vi "Kalman F.vi"(10 "Ball?":bool, 11 "intervalo":dbl) -> (1 "Q":T1, 2 "F'":T1, 3 "F":T1)   [LabVIEW 2017]
uses:
  <vilib>/Analysis/Matrix/Datatypes/RealMatrix.ctl
  <vilib>/Analysis/Matrix/Numeric/Multiply/Multiply - R,RM.vi
  <vilib>/Analysis/Matrix/Numeric/Add/Add - RM,RM.vi
  <vilib>/Analysis/Matrix/NI_Matrix.lvlib
  <vilib>/Analysis/Matrix/Numeric/Multiply/Multiply - RM,RM.vi
  <vilib>/Analysis/Matrix/Numeric/Conversions/Array To Matrix - RA2.vi
  <vilib>/Analysis/Matrix/Numeric/Conversions/Array To Matrix - RA.vi
  <vilib>/Analysis/Matrix/Numeric/Multiply/Multiply - RM,R.vi
panel:
  out "Real Matrix (Column Vector)":T1
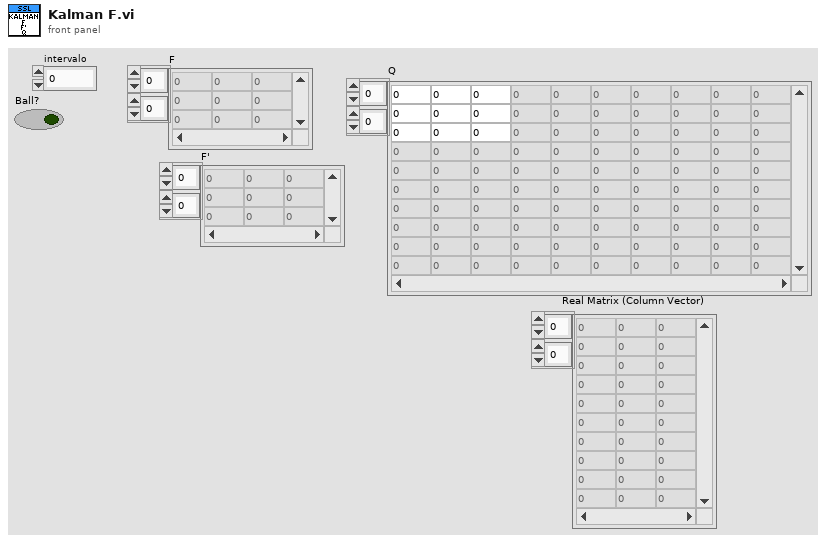
[diagram p1: front panel]
types:
  T1 = typedef "NI_Matrix.lvlib/RealMatrix.ctl" = dbl[][]
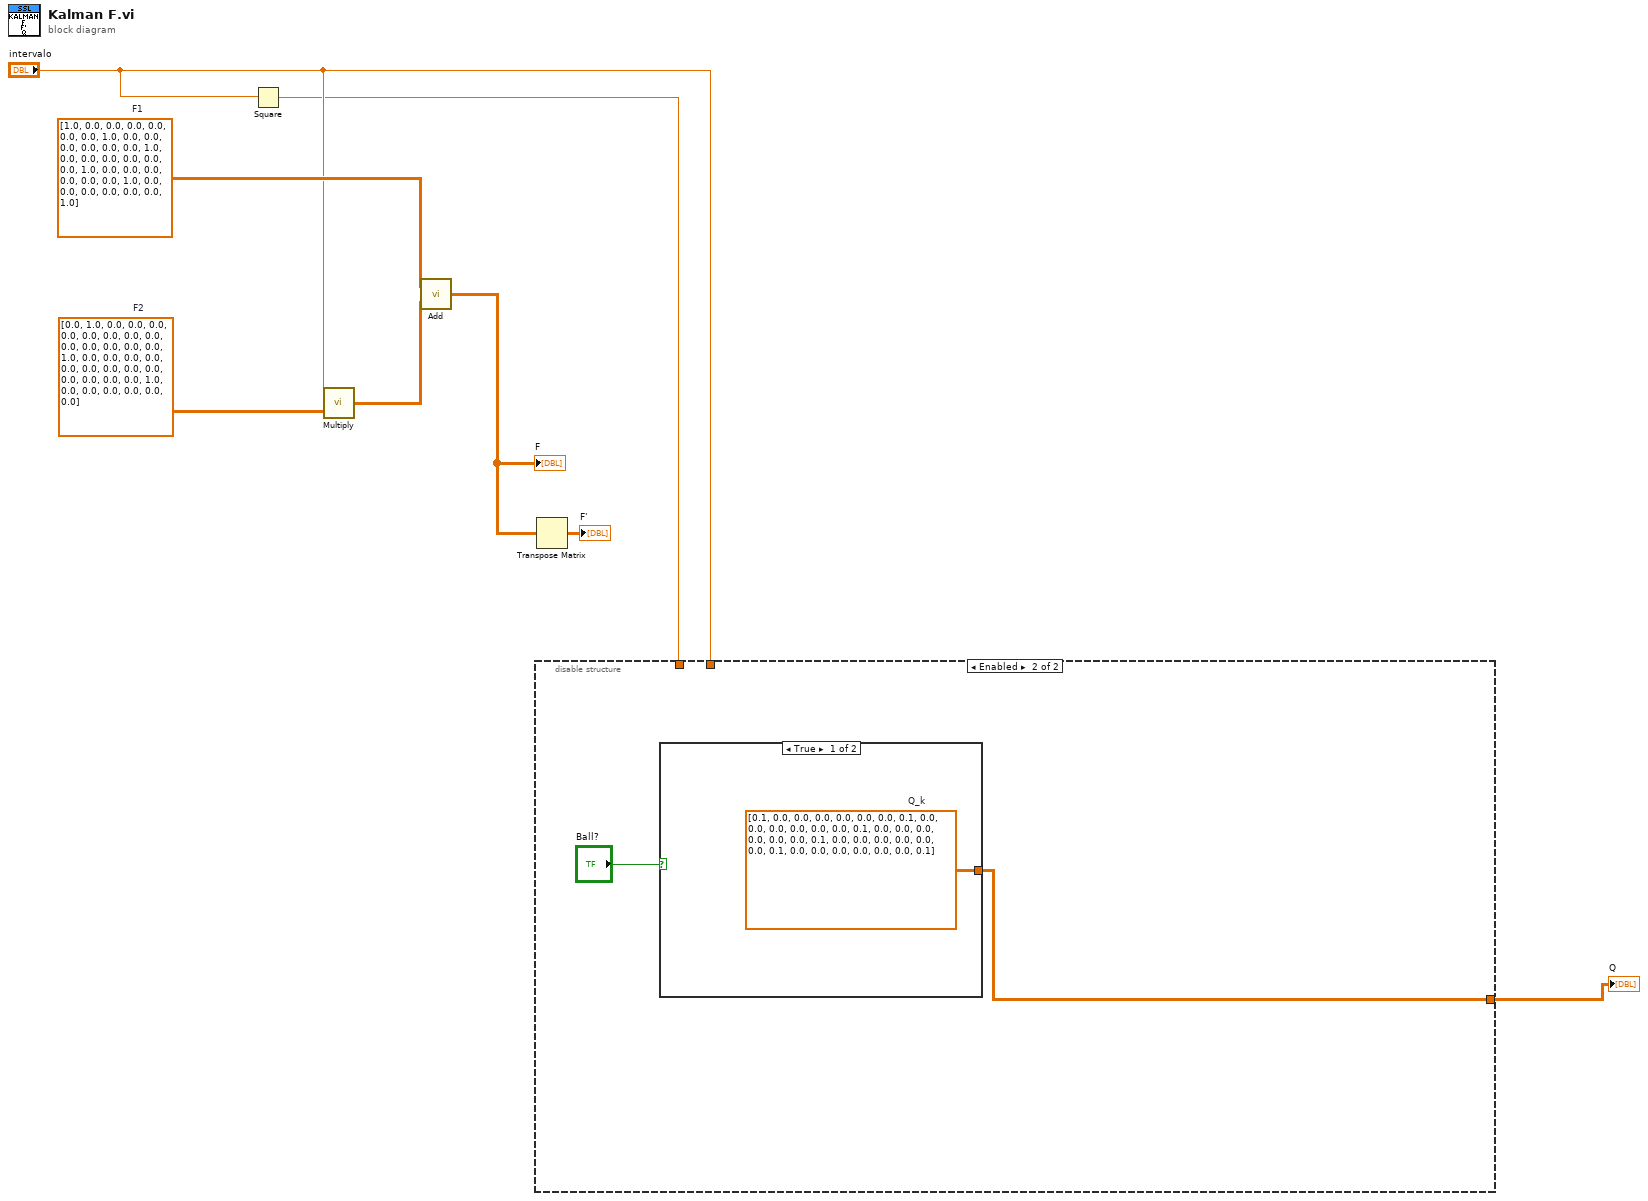
[diagram p0: block diagram]
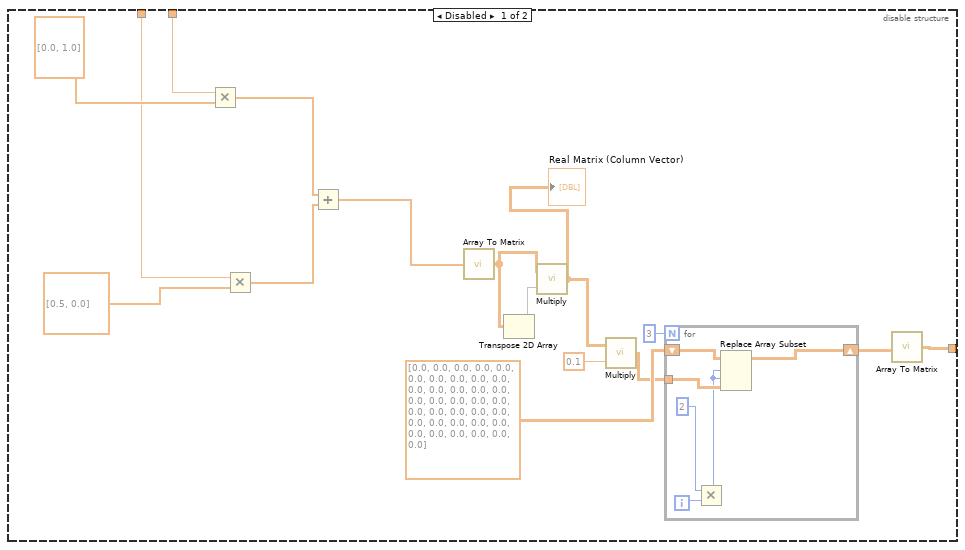
[diagram p2: hidden frame]
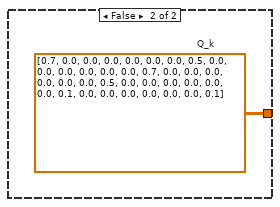
[diagram p3: hidden frame]
diagram:
  w6 = T1 [[0.0, 1.0, 0.0, 0.0, 0.0, 0.0], [0.0, 0.0, 0.0, 0.0, 0.0, 0.0], [0.0, 0.0, 0.0, 1.0, 0.0, 0.0], [0.0, 0.0, 0.0, 0.0, 0.0, 0.0], [0.0, 0.0, 0.0, 0.0, 0.0, 1.0], [0.0, 0.0, 0.0, 0.0, 0.0, 0.0]]  # F2
  w7 = T1 [[1.0, 0.0, 0.0, 0.0, 0.0, 0.0], [0.0, 1.0, 0.0, 0.0, 0.0, 0.0], [0.0, 0.0, 1.0, 0.0, 0.0, 0.0], [0.0, 0.0, 0.0, 1.0, 0.0, 0.0], [0.0, 0.0, 0.0, 0.0, 1.0, 0.0], [0.0, 0.0, 0.0, 0.0, 0.0, 1.0]]  # F1
  n1 = Square(x="intervalo") -> (x^2=w3:dbl)
  n2 = call-poly <vilib>:"Multiply.vi"("Real Matrix A"=w6, "Real Scalar c"="intervalo") -> ("c * A"=w8:T1)
  n3 = call-poly <vilib>:"Add.vi"("Real Matrix B"=w8, "Real Matrix A"=w7) -> ("A + B"=w2:T1)
  "F" <- w2
  n4 = disable-structure shown="Enabled" {
    disable-tunnel: "intervalo" -> [w24 _]
    disable-tunnel: w3 -> [w22 _]
    disable-tunnel: [w12 w32] -> w1
    frame Disabled {
      n5 = Multiply ("Multiply.vi")(x=w24, y=dbl[] [0.0, 1.0]) -> (x*y=w20:dbl[])
      n6 = Multiply ("Multiply.vi")(x=w22, y=dbl[] [0.5, 0.0]) -> (x*y=w19:dbl[])
      n7 = Add(x=w20, y=w19) -> (x+y=w18:dbl[])
      n8 = call-poly <vilib>:"Array To Matrix.vi"("Real 1D Array"=w18) -> ("Real Matrix (Column Vector)"=w16:T1)
      n9 = Transpose 2D Array(2D array=w16) -> (transposed array=w17:T1)
      n10 = call-poly <vilib>:"Multiply.vi"("Real Matrix B"=w17, "Real Matrix A"=w16) -> ("A * B"=w11:T1)
      "Real Matrix (Column Vector)" <- w11
      n11 = call-poly <vilib>:"Multiply.vi"("Real Scalar c"=0.1 ("y"), "Real Matrix A"=w11) -> ("A * c"=w10:T1)
      n12 = for {
        N: 3 -> [_]
        tunnel: w10 -> [w28]
        shift-right: [w27] -> w13
        shift-left: dbl[][] [[0.0, 0.0, 0.0, 0.0, 0.0, 0.0], [0.0, 0.0, 0.0, 0.0, 0.0, 0.0], [0.0, 0.0, 0.0, 0.0, 0.0, 0.0], [0.0, 0.0, 0.0, 0.0, 0.0, 0.0], [0.0, 0.0, 0.0, 0.0, 0.0, 0.0], [0.0, 0.0, 0.0, 0.0, 0.0, 0.0]] -> [w26]
        i -> [w30]
        n13 = Multiply(x=2, y=w30) -> (x*y=w25:i32)
        n14 = Replace Array Subset(array=w26, new element=w28, index (row)=w25, index (col)=w25) -> (w27:dbl[][])
      }
      n15 = call-poly <vilib>:"Array To Matrix.vi"("Real 2D Array"=w13) -> ("Real Matrix"=w12:T1)
    }
    frame Enabled {
      n16 = case shown="True" "Ball?" {
        tunnel: [w33 w34] -> w32
        frame True {
          w33 = T1 [[0.1, 0.0, 0.0, 0.0, 0.0, 0.0], [0.0, 0.1, 0.0, 0.0, 0.0, 0.0], [0.0, 0.0, 0.1, 0.0, 0.0, 0.0], [0.0, 0.0, 0.0, 0.1, 0.0, 0.0], [0.0, 0.0, 0.0, 0.0, 0.1, 0.0], [0.0, 0.0, 0.0, 0.0, 0.0, 0.1]]  # Q_k
        }
        frame False {
          w34 = T1 [[0.7, 0.0, 0.0, 0.0, 0.0, 0.0], [0.0, 0.5, 0.0, 0.0, 0.0, 0.0], [0.0, 0.0, 0.7, 0.0, 0.0, 0.0], [0.0, 0.0, 0.0, 0.5, 0.0, 0.0], [0.0, 0.0, 0.0, 0.0, 0.1, 0.0], [0.0, 0.0, 0.0, 0.0, 0.0, 0.1]]  # Q_k
        }
      }
    }
  }
  "Q" <- w1
  n17 = Transpose Matrix(1:w2) -> (0:→"F'":T1)
